vi "Replace Item(s) at Offset.vi"   [LabVIEW 2015, in "JSONtext.lvlib"]
uses:
  JSONtext.lvlib
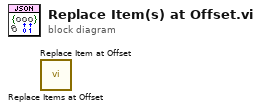
[diagram p0: block diagram]
diagram:
  n1 = call "Replace Items at Offset.vi"() -> ()  [unwired: 10 in, 2 out]
  n2 = call "Replace Item at Offset.vi"() -> ()  [unwired: 10 in, 2 out]
